vi "PJ1_ui-commu_1.vi"() -> ()   [LabVIEW 2024]
uses:
  contron/Control 7.ctl
  contron/Control 6.ctl
  contron/Control 5.ctl
  contron/Control 8.ctl
  contol_vr 23/66.ctl
  <vilib>/picture/picture.llb/imagedata.ctl
  contol_vr 23/Control 9.ctl
  contol_vr 23/6.ctl
  contol_vr 23/Control 4.ctl
  contol_vr 23/Control 3.ctl
  <vilib>/Instr/_visa.llb/VISA Configure Serial Port (Instr).vi
  <vilib>/express/express analysis/Spectral/Block/exnSpectralBlock spectral measurements PSD poly.vi
  <vilib>/express/express analysis/Spectral/Block/exnSpectralBlock spectral measurements PSD DDT.vi
  <vilib>/express/express analysis/Spectral/XNode/ExpressSpectralMeasurementsBlockNode.xnode
panel:
  out "check":bool
  out "Clear1":bool
  out "com":bool
  out "call":bool
  out "ele":bool
  in  "start":bool
  in  "Baseline":bool
  in  "VISA resource name":refnum<visa-resource-name>
  out "555":bool
  out "6 HZ 2":bool
  out "image data":T1
  out "7 HZ":bool
  in  "Upper Cut-Off":dbl=40.0
  out "PSD":dynamicdata(graph)
  out "PSD MAX":dbl
  out "Index ที่มากที่สุด":i32
  out "max value":dbl
  out "B 18+1":dbl
  out "N 18+1":dbl
  in  "Aj 18+1":dbl
  out "B 18+1":dbl
  out "PSD 18+1":dbl
  out "B 18":dbl
  out "N 18":dbl
  in  "Aj 18":dbl
  out "B 18":dbl
  out "PSD 18":dbl
  out "B 18-1":dbl
  out "N 18-1":dbl
  in  "Aj 18-1":dbl
  out "B 18-1":dbl
  out "PSD 18-1":dbl
  out "9 Hz":dbl[](array[numeric])
  out "Max Index 9":i32
  out "PSD max 9":dbl
  out "PSD 9-1":dbl
  out "B 9-1":dbl
  in  "Aj 9-1":dbl
  out "N 9-1":dbl
  out "B 9-1":dbl
  out "PSD 9":dbl
  out "B 9":dbl
  in  "Aj 9":dbl
  out "N 9":dbl
  out "B 9":dbl
  out "PSD 9+1":dbl
  out "B 9+1":dbl
  in  "Aj 9+1":dbl
  out "N 9+1":dbl
  out "B 9+1":dbl
  out "8 Hz":dbl[](array[numeric])
  out "Max Index 8":i32
  out "PSD max 8":dbl
  out "B 16+1":dbl
  out "N 16+1":dbl
  in  "Aj  16+1":dbl
  out "B 16+1":dbl
  out "PSD  16+1":dbl
  out "B 16":dbl
  out "N  16":dbl
  in  "Aj  16":dbl
  out "B 16":dbl
  out "PSD  16":dbl
  out "B 16-1":dbl
  out "N  16-1":dbl
  in  "Aj   16-1":dbl
  out "B   16-1":dbl
  out "PSD 16-1":dbl
  out "B 8+1":dbl
  out "N 8+1":dbl
  in  "Aj  8+1":dbl
  out "B  8+1":dbl
  out "PSD 8+1":dbl
  out "B 8":dbl
  out "N  8":dbl
  in  "Aj  8":dbl
  out "B  8":dbl
  out "PSD 8":dbl
  out "B 8-1":dbl
  out "N  8-1":dbl
  in  "Aj  8-1":dbl
  out "B  8-1":dbl
  out "PSD 8-1":dbl
  out "PSD 14+1":dbl
  out "B 14+1":dbl
  in  "Aj 14+1":dbl
  out "N 14+1":dbl
  out "B 14+1":dbl
  out "PSD 14":dbl
  out "B 14":dbl
  in  "Aj 14":dbl
  out "N 14":dbl
  out "B 14":dbl
  out "PSD 14-1":dbl
  out "B 14-1":dbl
  in  "Aj 14-1":dbl
  out "N 14-1":dbl
  out "B 14-1":dbl
  out "PSD7+1":dbl
  out "B7+1":dbl
  in  "Aj7+1":dbl
  out "N7+1":dbl
  out "B7+1":dbl
  out "PSD 7":dbl
  out "B 7":dbl
  in  "Aj 7":dbl
  out "N7":dbl
  out "B7":dbl
  out "7 Hz":dbl[](array[numeric])
  out "Max Index 7":i32
  out "PSD max 7":dbl
  out "PSD 7-1":dbl
  out "B 7-1":dbl
  in  "Aj 7-1":dbl
  out "N7-1":dbl
  out "B7-1":dbl
  out "B12-1":dbl
  out "N12-1":dbl
  in  "Aj 12-1":dbl
  out "B 12-1":dbl
  out "PSD 12-1":dbl
  out "B12":dbl
  out "N12":dbl
  in  "Aj 12":dbl
  out "B12":dbl
  out "PSD 12":dbl
  out "B12+1":dbl
  out "N12+1":dbl
  in  "Aj 12+1":dbl
  out "B 12+1":dbl
  out "PSD 12+1":dbl
  out "B6+1":dbl
  out "N6+1":dbl
  in  "Aj 6+1":dbl
  out "B 6+1":dbl
  out "PSD 6+1":dbl
  out "B6":dbl
  out "N6":dbl
  in  "Aj 6":dbl
  out "B6":dbl
  out "PSD 6":dbl
  out "PSD 6-1":dbl
  out "6 Hz":dbl[](array[numeric])
  out "Max Index 6":i32
  out "PSD max 6":dbl
  out "B 6-1":dbl
  in  "Aj 6-1":dbl
  out "N6-1":dbl
  out "B6-1":dbl
  out "appended array":dbl[][](array[numeric])
  out "Filtered Signal":dynamicdata(graph)
  in  "Lower Cut-Off":dbl=1.0
  out "data":dynamicdata(graph) caption="Raw Data"
  in  "number of samples":i32=1000
  in  "rate":dbl=200.0 min=200.0 max=200.0
  out "?":bool
  out "?":bool
  out "?":bool
  out "?":bool
  out "?":bool
  out "?":bool
  out "?":bool
  out "?":bool
  out "?":bool
  out "?":bool
  out "?":bool=TRUE
  out "?":bool=TRUE
  out "?":bool=TRUE
  out "?":bool=TRUE
  out "?":bool=TRUE
  out "?":bool=TRUE
  out "?":bool=TRUE
  out "?":bool=TRUE
  out "?":bool=TRUE
  out "?":bool=TRUE
  out "?":bool
  out "?":bool
  out "?":bool
  out "?":bool
  out "?":bool
  out "?":bool
  out "?":bool
  out "?":bool
  out "?":bool
  out "?":bool
  out "?":bool=TRUE
  out "?":bool=TRUE
  out "?":bool=TRUE
  out "?":bool=TRUE
  out "?":bool=TRUE
  out "?":bool=TRUE
  out "?":bool=TRUE
  out "?":bool=TRUE
  out "?":bool=TRUE
  out "?":bool=TRUE
  out "?":bool
  out "?":bool
  out "?":bool
  out "?":bool
  out "?":bool
  out "?":bool
  out "?":bool
  out "?":bool
  out "?":bool
  out "?":bool
  out "?":bool=TRUE
  out "?":bool=TRUE
  out "?":bool=TRUE
  out "?":bool=TRUE
  out "?":bool=TRUE
  out "?":bool=TRUE
  out "?":bool=TRUE
  out "?":bool=TRUE
  out "?":bool=TRUE
  out "?":bool=TRUE
  out "?":bool
  out "?":bool
  out "?":bool
  out "?":bool
  out "?":bool
  out "?":bool
  out "?":bool
  out "?":bool
  out "?":bool
  out "?":bool
  out "?":bool=TRUE
  out "?":bool=TRUE
  out "?":bool=TRUE
  out "?":bool=TRUE
  out "?":bool=TRUE
  out "?":bool=TRUE
  out "?":bool=TRUE
  out "?":bool=TRUE
  out "?":bool=TRUE
  out "?":bool=TRUE
  out "9 HZ":bool
  out "8 HZ":bool
  in  "Tab Control":T2(tab)
  out "Emotion 7":bool
  out "Emotion 6":bool
  out "Emotion 5":bool
  out "Emotion 4":bool
  out "ele":T3
  out "Emer":bool
  out "call":T4
  out "commu":T5
  in  "Activity":bool
  out "8-2":bool
  out "9-2":bool
  out "7-2":bool
  out "6-2":bool
  in  "Emotion":bool
  in  "ACC":T6
  in  "back_page2":T7
  in  "send":bool
  in  "BACK_Page3":bool
  out "Emotion 27":bool
  out "Emotion 26":bool
  out "Emotion 25":bool
  out "Emotion 24":bool
  in  "1 3":bool
  in  "1 2":T8
  in  "1":bool
  out "String 2":string
  in  "SOS CALLING":bool
  in  "Search Button 2":bool
  out "Emotion 15":bool
  out "Emotion 14":bool
  out "Emotion 13":bool
  out "Emotion 12":bool
  in  "Blank Button 14":bool
  in  "LED":bool
  in  "Blank Button 12":bool
  in  "BACK_Page4":bool
  out "BACK_page5":bool
  out "Emotion 3":bool
  out "Emotion 2":bool
  in  "BACK_Page5":bool=TRUE
  in  "Button 3":bool=TRUE
  in  "Button 2":bool=TRUE
  in  "Button 1":bool=TRUE
  out "Emotion 1":bool
  out "Emotion 11":bool
  in  "BACK_Page6":T9
  out "Emotion 10":bool
  out "Emotion 9":bool
  out "Emotion 8":bool
  in  "Activity 1":path
  out "new picture":picture
  in  "Activity 2":path
  in  "Activity 3":path
  out "new picture 2":picture
  out "new picture 3":picture
  out "Emotion 19":bool
  out "Emotion 18":bool
  out "Emotion 17":bool
  out "Emotion 16":bool
  out "new picture 7":picture
  in  "AAC13":path
  in  "Massage Send 3":string
  out "new picture 6":picture
  in  "AAC1 2":path
  in  "Massage Send 2":string
  out "new picture 5":picture
  in  "AAC1":path
  in  "BACK_Page7":bool
  in  "Massage Send 2":string
  out "Message Display":string
  in  "send 3":bool
  in  "Message Send":string
  in  "Clearpage 2":bool
  in  "Text3":T10
  in  "Text2":T11
  in  "Text1":bool
  in  "send 2":bool
  # "MENU"
  # "COMMUNICATION"
  # "SOS CALLING"
  # "Tel."
  # "ELECTRICAL DEVICES"
  # "EMOTIONS"
  # "ACTIVITIES"
  # "AAC"
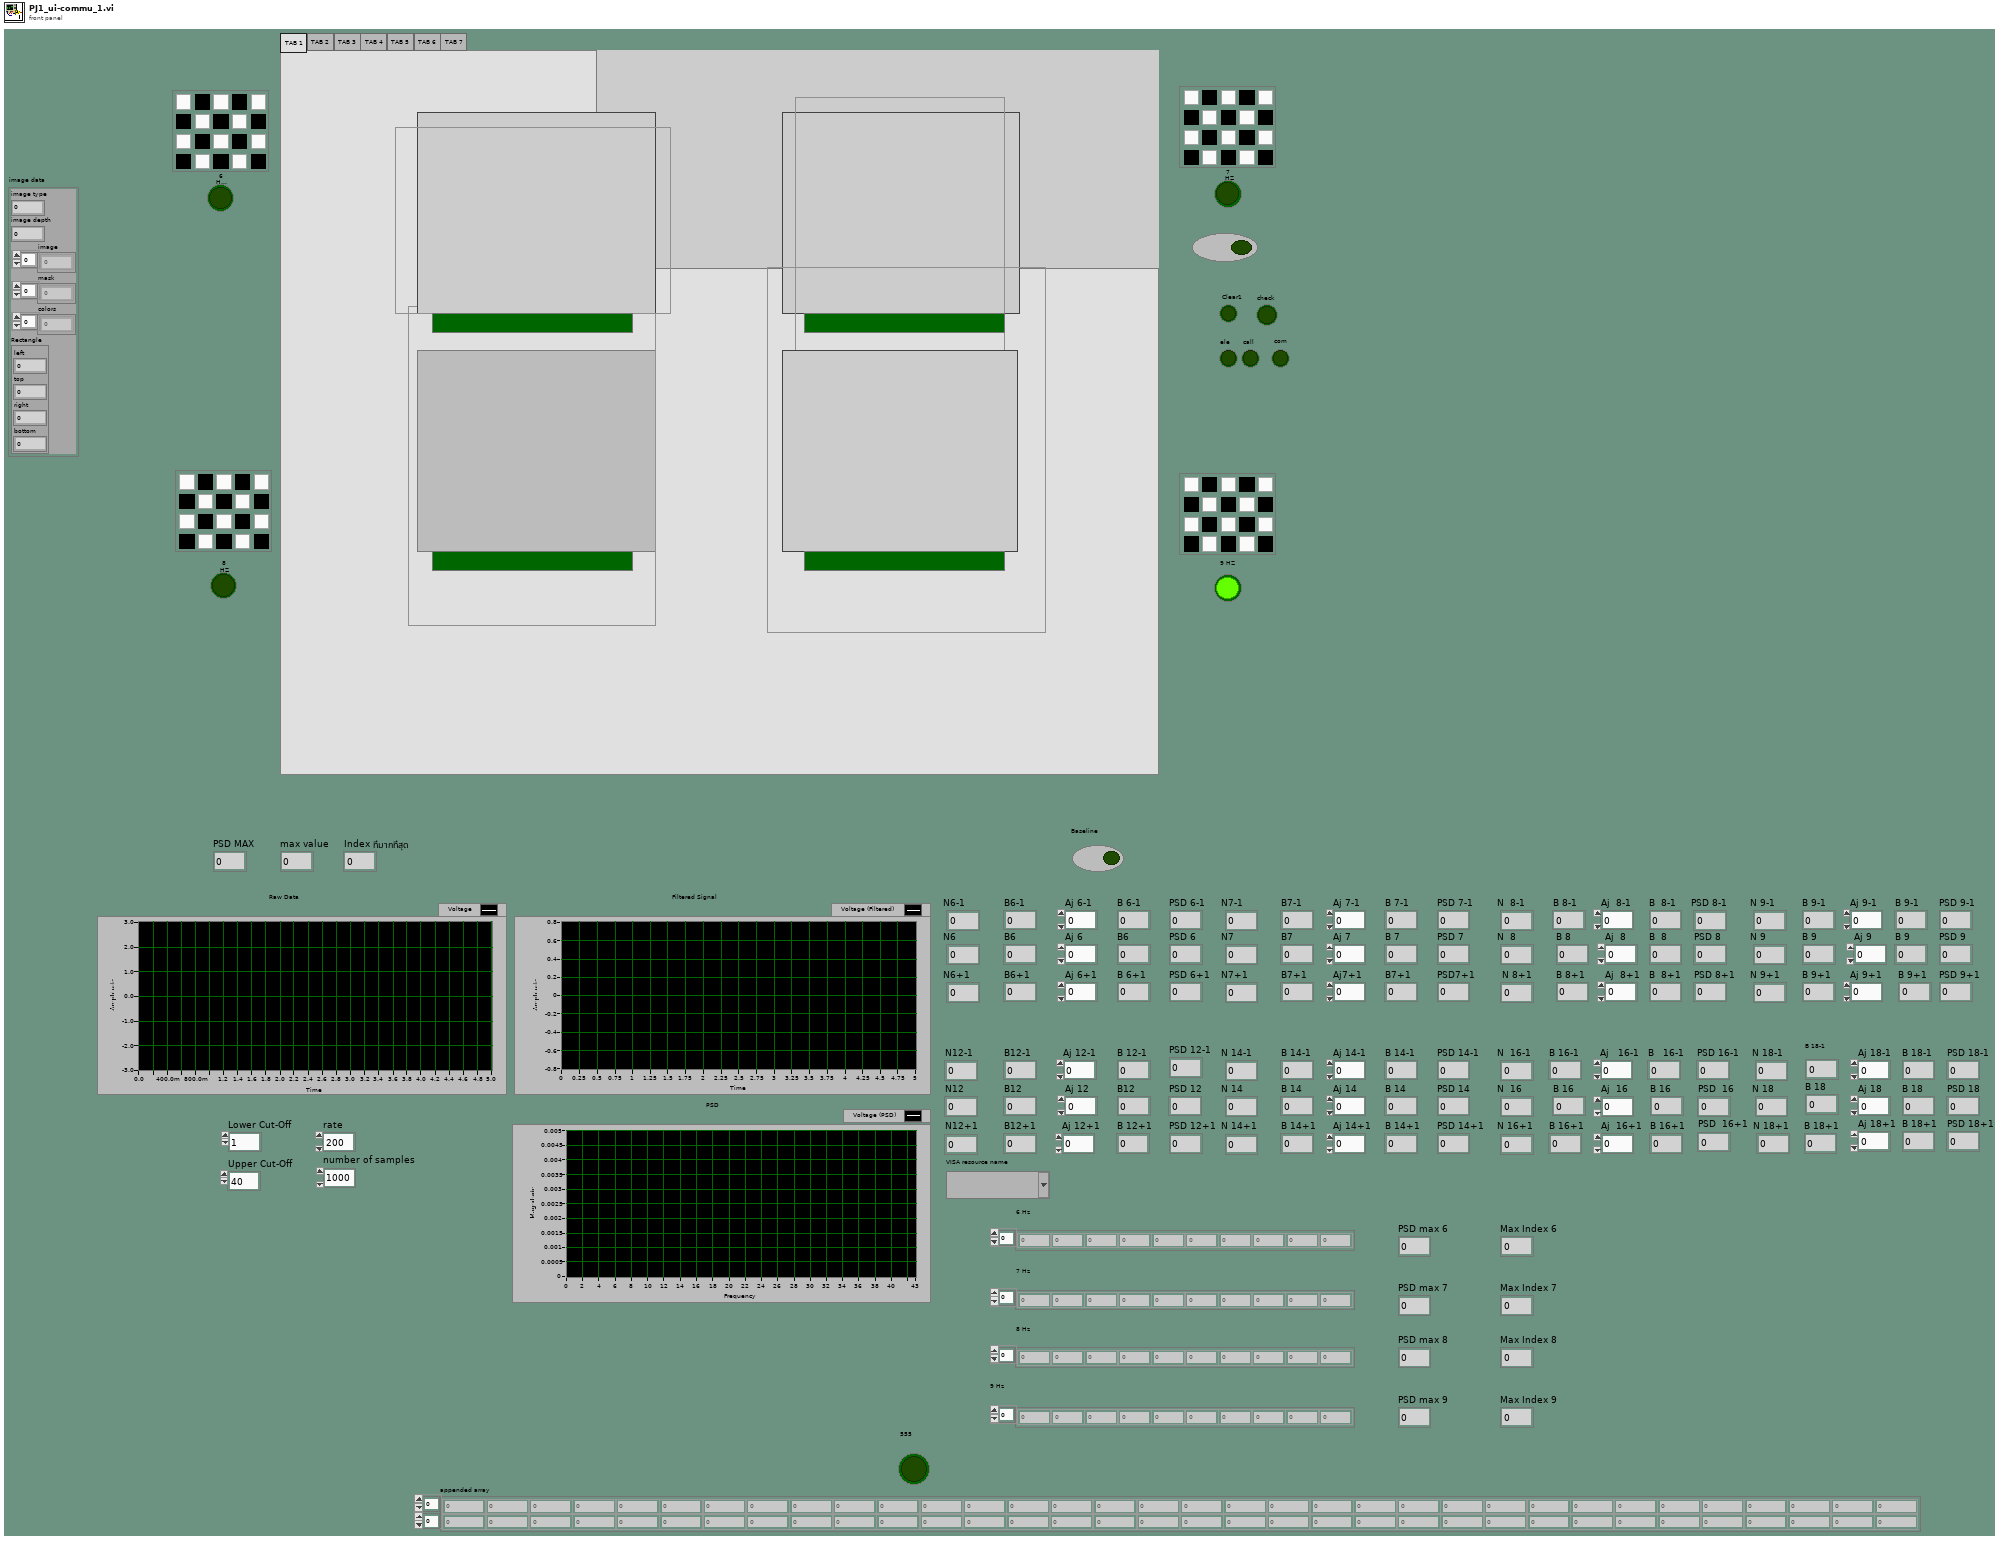
[diagram p1: front panel]
types:
  T1 = typedef "imagedata.ctl" = cluster{"image type":i32, "image depth":i32, "image":u8[], "mask":u8[], "colors":u32[], "Rectangle":cluster{"left":i16, "top":i16, "right":i16, "bottom":i16}}
  T2 = enum32{"TAB 1", "TAB 2", "TAB 3", "TAB 4", "TAB 5", "TAB 6", "TAB 7"}
  T3 = typedef "Control 5.ctl" = bool
  T4 = typedef "Control 6.ctl" = bool
  T5 = typedef "Control 7.ctl" = bool
  T6 = typedef "6.ctl" = bool
  T7 = typedef "66.ctl" = bool
  T8 = typedef "Control 8.ctl" = bool
  T9 = typedef "Control 9.ctl" = bool
  T10 = typedef "Control 4.ctl" = bool
  T11 = typedef "Control 3.ctl" = bool
  T12 = cluster{"averaging mode":u16, "weighting mode":u16, "number of averages":u32}
  T13 = cluster{"dB On (F)":bool, "unwrap phase (F)":bool, "convert to degree (F)":bool}
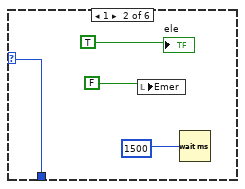
[diagram p2: hidden frame]
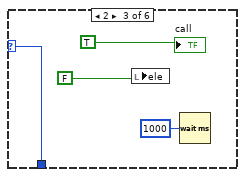
[diagram p3: hidden frame]
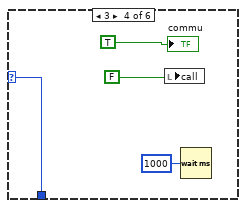
[diagram p4: hidden frame]
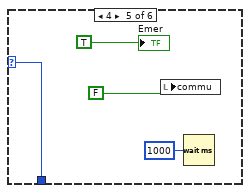
[diagram p5: hidden frame]
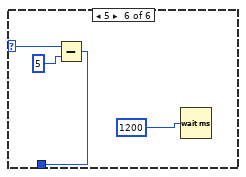
[diagram p6: hidden frame]
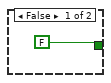
[diagram p8: hidden frame]
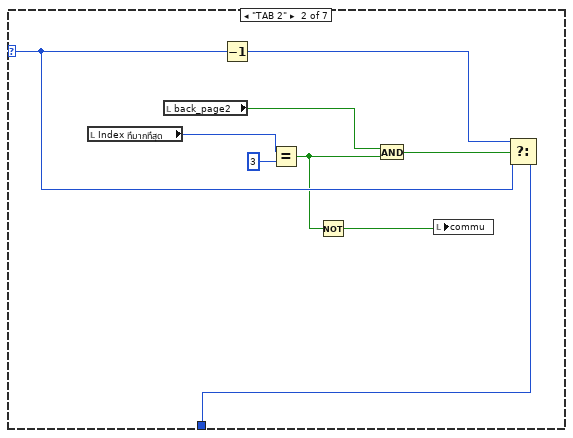
[diagram p9: hidden frame]
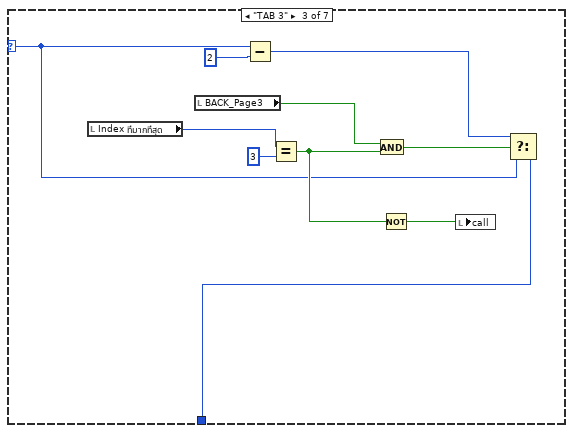
[diagram p10: hidden frame]
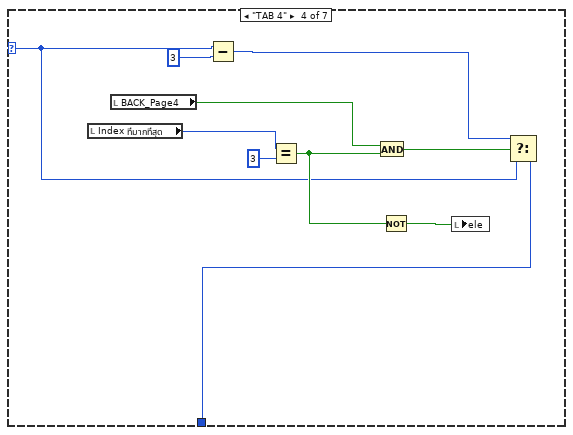
[diagram p11: hidden frame]
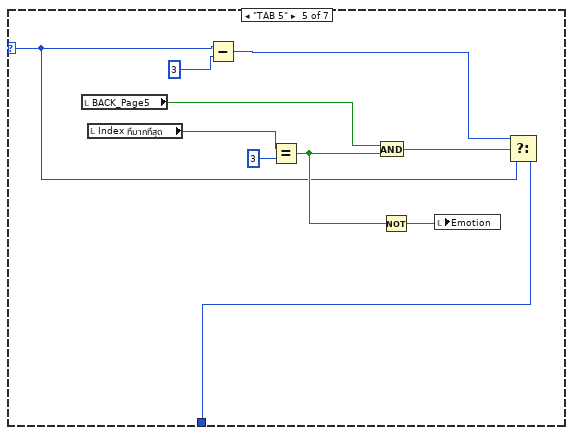
[diagram p12: hidden frame]
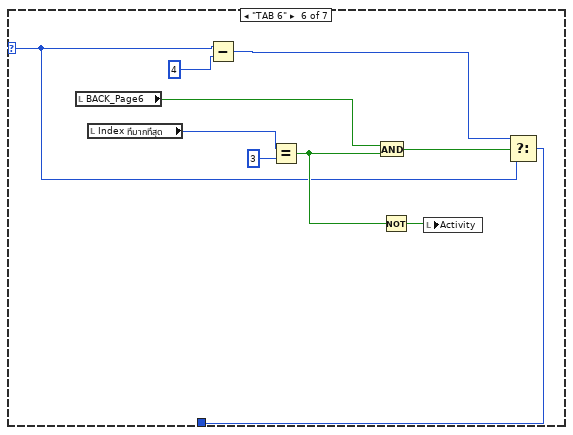
[diagram p13: hidden frame]
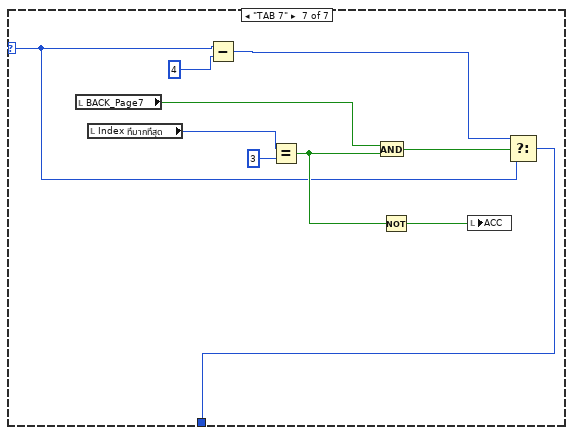
[diagram p14: hidden frame]
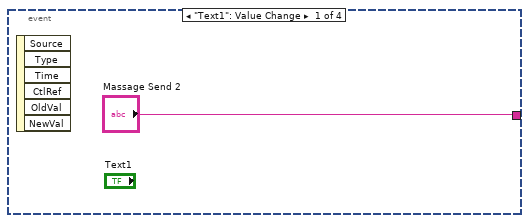
[diagram p15: hidden frame]
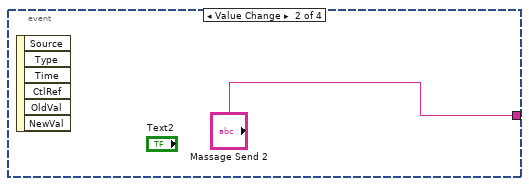
[diagram p16: hidden frame]
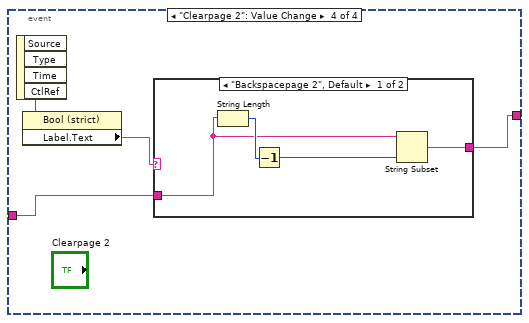
[diagram p17: hidden frame]
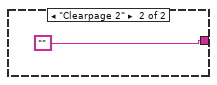
[diagram p18: hidden frame]
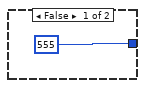
[diagram p19: hidden frame]
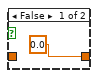
[diagram p20: hidden frame]
diagram:
  n1 = while {
    shift-right: [w23] -> _
    shift-left: "" -> [w25]
    stop <- FALSE stop-if-true
    n2 = event shown="[3] \"BACK_Page3\": Value Change" {
      selector: _ -> [_ _ _ _]
      dyn-events: _ -> [_ _ _ _]
      timeout: _ -> [_ _ _ _]
      tunnel: w25 -> [_ _ _ _]
      tunnel: ["0622436287" "1669" " 0937529340" _] -> w23
      event Value Change {
        n3 = event-data() -> ()  [unwired: 1 in, 6 out]
      }
      event "1": Value Change {
        n4 = event-data() -> ()  [unwired: 1 in, 6 out]
      }
      event "1 3": Value Change {
        n5 = event-data() -> ()  [unwired: 1 in, 6 out]
      }
      event "BACK_Page3": Value Change {
        n6 = event-data() -> ()  [unwired: 1 in, 6 out]
        n7 = local write "Tab Control"(enum32{"TAB 1", "TAB 2", "TAB 3", "TAB 4"}."TAB 1" ("Tab Control")) -> ()
      }
    }
    "String 2" <- w23
  }
  n8 = while {
    stop <- FALSE stop-if-true
    n9 = while {
      stop <- FALSE stop-if-true
      n10 = while {
        stop <- FALSE stop-if-true
        w69 = 83.3333
        # "6 HZ"
        n11 = for {
          N: 2 -> [_]
          tunnel: w69 -> [w73]
          i -> [w75]
          n12 = Wait (ms)(milliseconds to wait=w73) -> ()  [unwired: 1 out]
          n13 = Equal?(x=0, y=w75) -> (x = y?=→"?" →"?" →"?" →"?" →"?" →"?" →"?" →"?" →"?" →"?":bool)
        }
        n14 = for {
          N: 2 -> [_]
          tunnel: w69 -> [w77]
          i -> [w78]
          n15 = Wait (ms)(milliseconds to wait=w77) -> ()  [unwired: 1 out]
          n16 = Equal?(x=1, y=w78) -> (x = y?=→"?" →"?" →"?" →"?" →"?" →"?" →"?" →"?" →"?" →"?":bool)
        }
      }
      n17 = while {
        stop <- FALSE stop-if-true
        w57 = 71.428571
        # "7 HZ"
        n18 = for {
          N: 2 -> [_]
          tunnel: w57 -> [w61]
          i -> [w63]
          n19 = Wait (ms)(milliseconds to wait=w61) -> ()  [unwired: 1 out]
          n20 = Equal?(x=0, y=w63) -> (x = y?=→"?" →"?" →"?" →"?" →"?" →"?" →"?" →"?" →"?" →"?":bool)
        }
        n21 = for {
          N: 2 -> [_]
          tunnel: w57 -> [w65]
          i -> [w66]
          n22 = Wait (ms)(milliseconds to wait=w65) -> ()  [unwired: 1 out]
          n23 = Equal?(x=1, y=w66) -> (x = y?=→"?" →"?" →"?" →"?" →"?" →"?" →"?" →"?" →"?" →"?":bool)
        }
      }
      n24 = while {
        stop <- FALSE stop-if-true
        w45 = 62.5
        # "8 HZ"
        n25 = for {
          N: 2 -> [_]
          tunnel: w45 -> [w49]
          i -> [w51]
          n26 = Wait (ms)(milliseconds to wait=w49) -> ()  [unwired: 1 out]
          n27 = Equal?(x=0, y=w51) -> (x = y?=→"?" →"?" →"?" →"?" →"?" →"?" →"?" →"?" →"?" →"?":bool)
        }
        n28 = for {
          N: 2 -> [_]
          tunnel: w45 -> [w53]
          i -> [w54]
          n29 = Wait (ms)(milliseconds to wait=w53) -> ()  [unwired: 1 out]
          n30 = Equal?(x=1, y=w54) -> (x = y?=→"?" →"?" →"?" →"?" →"?" →"?" →"?" →"?" →"?" →"?":bool)
        }
      }
      n31 = while {
        stop <- FALSE stop-if-true
        w33 = 55.5555
        # "9 HZ"
        n32 = for {
          N: 2 -> [_]
          tunnel: w33 -> [w37]
          i -> [w39]
          n33 = Wait (ms)(milliseconds to wait=w37) -> ()  [unwired: 1 out]
          n34 = Equal?(x=0, y=w39) -> (x = y?=→"?" →"?" →"?" →"?" →"?" →"?" →"?" →"?" →"?" →"?":bool)
        }
        n35 = for {
          N: 2 -> [_]
          tunnel: w33 -> [w41]
          i -> [w42]
          n36 = Wait (ms)(milliseconds to wait=w41) -> ()  [unwired: 1 out]
          n37 = Equal?(x=1, y=w42) -> (x = y?=→"?" →"?" →"?" →"?" →"?" →"?" →"?" →"?" →"?" →"?":bool)
        }
      }
    }
  }
  n38 = while {
    stop <- FALSE stop-if-true
    n39 = call "DAQ Assistant2"("rate"="rate", "number of samples"="number of samples") -> ("data"=w84:dynamicdata)  [unwired: 15 in, 2 out]
    "data" <- w84
    n40 = Divide(x="rate", y="number of samples") -> (x/y=w171:dbl)
    n41 = call "Filter"("Lower Cut-Off"="Lower Cut-Off", "Upper Cut-Off"="Upper Cut-Off", "Signal"=w84) -> ("Filtered Signal"=w85:dynamicdata)  [unwired: 7 in, 1 out]
    "Filtered Signal" <- w85
    n42 = Divide(x=8.0, y=w171) -> (x/y=w271:dbl)
    n43 = Divide(x=16.0, y=w171) -> (x/y=w223:dbl)
    n44 = Divide(x=14.0, y=w171) -> (x/y=w296:dbl)
    n45 = Divide(x=18.0, y=w171) -> (x/y=w146:dbl)
    n46 = xnode "Spectral Measurements"("Signals"=w85) -> ("PSD"=w111:dynamicdata)  [unwired: 1 in, 1 out]
    "PSD" <- w111
    n47 = Divide(x=9.0, y=w171) -> (x/y=w189:dbl)
    n48 = Divide(x=7.0, y=w171) -> (x/y=w313:dbl)
    n49 = Divide(x=12.0, y=w171) -> (x/y=w382:dbl)
    n50 = Divide(x=6.0, y=w171) -> (x/y=w431:dbl)
    n51 = call "Convert from Dynamic Data"("Dynamic Data Type"=w111) -> ("Array"=w461:dbl[])  [unwired: 3 in]
    n52 = Decrement(x=w189) -> (x-1=w220:dbl)
    n53 = Increment(x=w189) -> (x+1=w188:dbl)
    n54 = Increment(x=w146) -> (x+1=w135:dbl)
    n55 = Decrement(x=w146) -> (x-1=w160:dbl)
    n56 = Decrement(x=w296) -> (x-1=w325:dbl)
    n57 = Increment(x=w271) -> (x+1=w261:dbl)
    n58 = Decrement(x=w223) -> (x-1=w246:dbl)
    n59 = Decrement(x=w431) -> (x-1=w444:dbl)
    n60 = Decrement(x=w313) -> (x-1=w354:dbl)
    "PSD 7-1" <- w354
    n61 = Increment(x=w313) -> (x+1=w339:dbl)
    n62 = Decrement(x=w271) -> (x-1=w284:dbl)
    n63 = Increment(x=w223) -> (x+1=w222:dbl)
    n64 = Increment(x=w431) -> (x+1=w420:dbl)
    n65 = Increment(x=w296) -> (x+1=w302:dbl)
    n66 = Decrement(x=w382) -> (x-1=w387:dbl)
    n67 = Increment(x=w382) -> (x+1=w381:dbl)
    n68 = Build Array(w461) -> (w136:dbl[][])
    "appended array" <- w136
    n69 = Index Array(array=w136, index (row)=0, index (col)=w246) -> (element=w257:dbl)
    "PSD 16-1" <- w257
    n70 = Index Array(array=w136, index (row)=0 ("disabled index (row)"), index (col)=w222) -> (element=w234:dbl)
    "PSD  16+1" <- w234
    n71 = Index Array(array=w136, index (row)=0 ("disabled index (row)"), index (col)=w223) -> (element=w236:dbl)
    "PSD  16" <- w236
    n72 = Index Array(array=w136, index (row)=0, index (col)=w302) -> (element=w303:dbl)
    "PSD 14+1" <- w303
    n73 = Index Array(array=w136, index (row)=0 ("disabled index (row)"), index (col)=w160) -> (element=w158:dbl)
    "PSD 18-1" <- w158
    n74 = Index Array(array=w136, index (row)=0, index (col)=w261) -> (element=w259:dbl)
    "PSD 8+1" <- w259
    n75 = Index Array(array=w136, index (row)=0 ("disabled index (row)"), index (col)=w135) -> (element=w132:dbl)
    "PSD 18+1" <- w132
    n76 = Index Array(array=w136, index (row)=0, index (col)=w188) -> (element=w177:dbl)
    "PSD 9-1" <- w177
    n77 = Index Array(array=w136, index (row)=0, index (col)=w271) -> (element=w282:dbl)
    "PSD 8" <- w282
    n78 = Index Array(array=w136, index (row)=0 ("disabled index (row)"), index (col)=w146) -> (element=w147:dbl)
    "PSD 18" <- w147
    n79 = Index Array(array=w136, index (row)=0, index (col)=w284) -> (element=w283:dbl)
    "PSD 8-1" <- w283
    n80 = Index Array(array=w136, index (row)=0, index (col)=w189) -> (element=w190:dbl)
    "PSD 9" <- w190
    n81 = Index Array(array=w136, index (row)=0, index (col)=w220) -> (element=w201:dbl)
    "PSD 9+1" <- w201
    n82 = Index Array(array=w136, index (row)=0, index (col)=w325) -> (element=w327:dbl)
    "PSD 14-1" <- w327
    n83 = Index Array(array=w136, index (row)=0, index (col)=w296) -> (element=w314:dbl)
    "PSD 14" <- w314
    n84 = Index Array(array=w136, index (row)=0, index (col)=w354) -> ()  [unwired: 1 out]
    n85 = Index Array(array=w136, index (row)=0 ("disabled index (row)"), index (col)=w313) -> (element=w351:dbl)
    "PSD 7" <- w351
    n86 = Index Array(array=w136, index (row)=0, index (col)=w339) -> (element=w340:dbl)
    "PSD7+1" <- w340
    n87 = Index Array(array=w136, index (row)=0 ("disabled index (row)"), index (col)=w420) -> (element=w418:dbl)
    "PSD 6+1" <- w418
    n88 = Index Array(array=w136, index (row)=0, index (col)=w387) -> (element=w386:dbl)
    "PSD 12-1" <- w386
    n89 = Index Array(array=w136, index (row)=0 ("disabled index (row)"), index (col)=w382) -> (element=w383:dbl)
    "PSD 12" <- w383
    n90 = Index Array(array=w136, index (row)=0 ("disabled index (row)"), index (col)=w381) -> (element=w379:dbl)
    "PSD 12+1" <- w379
    n91 = Index Array(array=w136, index (row)=0, index (col)=w431) -> (element=w432:dbl)
    "PSD 6" <- w432
    n92 = Index Array(array=w136, index (row)=0, index (col)=w444) -> (element=w451:dbl)
    "PSD 6-1" <- w451
    n93 = feedback #1() -> (w87:dbl)  [unwired: 1 in]
    "B 18" <- w87
    n94 = case shown="False" "Baseline" {
      tunnel: w147 -> [_ w472]
      tunnel: [w471 w472] -> w149
      tunnel: w87 -> [w471 _]
      frame False {
      }
      frame True {
      }
    }
    n95 = feedback-in #1(w149) -> ()
    n96 = feedback #2() -> (w88:dbl)  [unwired: 1 in]
    "B 18-1" <- w88
    n97 = case shown="False" "Baseline" {
      tunnel: w158 -> [_ w476]
      tunnel: [w475 w476] -> w169
      tunnel: w88 -> [w475 _]
      frame False {
      }
      frame True {
      }
    }
    n98 = feedback-in #2(w169) -> ()
    n99 = feedback #3() -> (w86:dbl)  [unwired: 1 in]
    "B 18+1" <- w86
    n100 = case shown="False" "Baseline" {
      tunnel: w132 -> [_ w468]
      tunnel: [w467 w468] -> w145
      tunnel: w86 -> [w467 _]
      frame False {
      }
      frame True {
      }
    }
    n101 = feedback-in #3(w145) -> ()
    n102 = feedback #4() -> (w94:dbl)  [unwired: 1 in]
    "B 16-1" <- w94
    n103 = case shown="True" "Baseline" {
      tunnel: w257 -> [_ w500]
      tunnel: [w499 w500] -> w247
      tunnel: w94 -> [w499 _]
      frame False {
      }
      frame True {
      }
    }
    n104 = feedback-in #4(w247) -> ()
    n105 = feedback #5() -> (w92:dbl)  [unwired: 1 in]
    "B 16+1" <- w92
    n106 = case shown="True" "Baseline" {
      tunnel: w234 -> [_ w492]
      tunnel: [w491 w492] -> w225
      tunnel: w92 -> [w491 _]
      frame False {
      }
      frame True {
      }
    }
    n107 = feedback-in #5(w225) -> ()
    n108 = feedback #6() -> (w93:dbl)  [unwired: 1 in]
    "B 16" <- w93
    n109 = case shown="True" "Baseline" {
      tunnel: w236 -> [_ w496]
      tunnel: [w495 w496] -> w245
      tunnel: w93 -> [w495 _]
      frame False {
      }
      frame True {
      }
    }
    n110 = feedback-in #6(w245) -> ()
    n111 = feedback #7() -> (w95:dbl)  [unwired: 1 in]
    "B 8+1" <- w95
    n112 = case shown="True" "Baseline" {
      tunnel: w259 -> [_ w504]
      tunnel: [w503 w504] -> w270
      tunnel: w95 -> [w503 _]
      frame False {
      }
      frame True {
      }
    }
    n113 = feedback-in #7(w270) -> ()
    n114 = feedback #8() -> (w98:dbl)  [unwired: 1 in]
    "B 14+1" <- w98
    n115 = case shown="True" "Baseline" {
      tunnel: w303 -> [_ w516]
      tunnel: [w515 w516] -> w304
      tunnel: w98 -> [w515 _]
      frame False {
      }
      frame True {
      }
    }
    n116 = feedback-in #8(w304) -> ()
    n117 = feedback #9() -> (w96:dbl)  [unwired: 1 in]
    "B 8" <- w96
    n118 = case shown="True" "Baseline" {
      tunnel: w282 -> [_ w508]
      tunnel: [w507 w508] -> w273
      tunnel: w96 -> [w507 _]
      frame False {
      }
      frame True {
      }
    }
    n119 = feedback-in #9(w273) -> ()
    n120 = feedback #10() -> (w90:dbl)  [unwired: 1 in]
    "B 9" <- w90
    n121 = case shown="False" "Baseline" {
      tunnel: w190 -> [_ w484]
      tunnel: [w483 w484] -> w191
      tunnel: w90 -> [w483 _]
      frame False {
      }
      frame True {
      }
    }
    n122 = feedback-in #10(w191) -> ()
    n123 = feedback #11() -> (w97:dbl)  [unwired: 1 in]
    "B 8-1" <- w97
    n124 = case shown="True" "Baseline" {
      tunnel: w283 -> [_ w512]
      tunnel: [w511 w512] -> w294
      tunnel: w97 -> [w511 _]
      frame False {
      }
      frame True {
      }
    }
    n125 = feedback-in #11(w294) -> ()
    n126 = feedback #12() -> (w91:dbl)  [unwired: 1 in]
    "B 9+1" <- w91
    n127 = case shown="True" "Baseline" {
      tunnel: w201 -> [_ w488]
      tunnel: [w487 w488] -> w202
      tunnel: w91 -> [w487 _]
      frame False {
      }
      frame True {
      }
    }
    n128 = feedback-in #12(w202) -> ()
    n129 = feedback #13() -> (w106:dbl)  [unwired: 1 in]
    "B12-1" <- w106
    n130 = case shown="True" "Baseline" {
      tunnel: w386 -> [_ w548]
      tunnel: [w547 w548] -> w398
      tunnel: w106 -> [w547 _]
      frame False {
      }
      frame True {
      }
    }
    n131 = feedback-in #13(w398) -> ()
    n132 = feedback #14() -> (w100:dbl)  [unwired: 1 in]
    "B 14-1" <- w100
    n133 = case shown="True" "Baseline" {
      tunnel: w327 -> [_ w524]
      tunnel: [w523 w524] -> w328
      tunnel: w100 -> [w523 _]
      frame False {
      }
      frame True {
      }
    }
    n134 = feedback-in #14(w328) -> ()
    n135 = feedback #15() -> (w89:dbl)  [unwired: 1 in]
    "B 9-1" <- w89
    n136 = case shown="False" "Baseline" {
      tunnel: w177 -> [_ w480]
      tunnel: [w479 w480] -> w178
      tunnel: w89 -> [w479 _]
      frame False {
      }
      frame True {
      }
    }
    n137 = feedback-in #15(w178) -> ()
    n138 = feedback #16() -> (w107:dbl)  [unwired: 1 in]
    "B6+1" <- w107
    n139 = case shown="True" "Baseline" {
      tunnel: w418 -> [_ w552]
      tunnel: [w551 w552] -> w421
      tunnel: w107 -> [w551 _]
      frame False {
      }
      frame True {
      }
    }
    n140 = feedback-in #16(w421) -> ()
    n141 = feedback #17() -> (w108:dbl)  [unwired: 1 in]
    "B6" <- w108
    n142 = case shown="True" "Baseline" {
      tunnel: w432 -> [_ w556]
      tunnel: [w555 w556] -> w442
      tunnel: w108 -> [w555 _]
      frame False {
      }
      frame True {
      }
    }
    n143 = feedback-in #17(w442) -> ()
    n144 = feedback #18() -> (w109:dbl)  [unwired: 1 in]
    "B6-1" <- w109
    n145 = case shown="False" "Baseline" {
      tunnel: w451 -> [_ w560]
      tunnel: [w559 w560] -> w443
      tunnel: w109 -> [w559 _]
      frame False {
      }
      frame True {
      }
    }
    n146 = feedback-in #18(w443) -> ()
    n147 = feedback #19() -> (w99:dbl)  [unwired: 1 in]
    "B 14" <- w99
    n148 = case shown="True" "Baseline" {
      tunnel: w314 -> [_ w520]
      tunnel: [w519 w520] -> w316
      tunnel: w99 -> [w519 _]
      frame False {
      }
      frame True {
      }
    }
    n149 = feedback-in #19(w316) -> ()
    n150 = feedback #20() -> (w104:dbl)  [unwired: 1 in]
    "B12+1" <- w104
    n151 = case shown="True" "Baseline" {
      tunnel: w379 -> [_ w540]
      tunnel: [w539 w540] -> w416
      tunnel: w104 -> [w539 _]
      frame False {
      }
      frame True {
      }
    }
    n152 = feedback-in #20(w416) -> ()
    n153 = Add(x=w87, y="Aj 18") -> (x+y=w153:dbl)
    "B 18" <- w153
    n154 = Add(x=w88, y="Aj 18-1") -> (x+y=w165:dbl)
    "B 18-1" <- w165
    n155 = Add(x=w86, y="Aj 18+1") -> (x+y=w141:dbl)
    "B 18+1" <- w141
    n156 = feedback #21() -> (w105:dbl)  [unwired: 1 in]
    "B12" <- w105
    n157 = case shown="True" "Baseline" {
      tunnel: w383 -> [_ w544]
      tunnel: [w543 w544] -> w399
      tunnel: w105 -> [w543 _]
      frame False {
      }
      frame True {
      }
    }
    n158 = feedback-in #21(w399) -> ()
    n159 = Add(x=w94, y="Aj   16-1") -> (x+y=w251:dbl)
    "B   16-1" <- w251
    n160 = Add(x=w92, y="Aj  16+1") -> (x+y=w229:dbl)
    "B 16+1" <- w229
    n161 = Add(x=w93, y="Aj  16") -> (x+y=w241:dbl)
    "B 16" <- w241
    n162 = Add(x=w95, y="Aj  8+1") -> (x+y=w266:dbl)
    "B  8+1" <- w266
    n163 = Add(x=w98, y="Aj 14+1") -> (x+y=w308:dbl)
    "B 14+1" <- w308
    n164 = Add(x=w96, y="Aj  8") -> (x+y=w277:dbl)
    "B  8" <- w277
    n165 = Add(x=w90, y="Aj 9") -> (x+y=w195:dbl)
    "B 9" <- w195
    n166 = Add(x=w97, y="Aj  8-1") -> (x+y=w290:dbl)
    "B  8-1" <- w290
    n167 = Add(x=w91, y="Aj 9+1") -> (x+y=w206:dbl)
    "B 9+1" <- w206
    n168 = Add(x=w106, y="Aj 12-1") -> (x+y=w394:dbl)
    "B 12-1" <- w394
    n169 = Add(x=w100, y="Aj 14-1") -> (x+y=w332:dbl)
    "B 14-1" <- w332
    n170 = Add(x=w89, y="Aj 9-1") -> (x+y=w182:dbl)
    "B 9-1" <- w182
    n171 = Multiply(x=w87, y=5.0) -> (x*y=w156:dbl)
    "N 18" <- w156
    n172 = Add(x=w107, y="Aj 6+1") -> (x+y=w425:dbl)
    "B 6+1" <- w425
    n173 = Multiply(x=w88, y=5.0) -> (x*y=w162:dbl)
    "N 18-1" <- w162
    n174 = Multiply(x=w86, y=5.0) -> (x*y=w138:dbl)
    "N 18+1" <- w138
    n175 = feedback #22() -> (w101:dbl)  [unwired: 1 in]
    "B7+1" <- w101
    n176 = case shown="True" "Baseline" {
      tunnel: w340 -> [_ w528]
      tunnel: [w527 w528] -> w342
      tunnel: w101 -> [w527 _]
      frame False {
      }
      frame True {
      }
    }
    n177 = feedback-in #22(w342) -> ()
    n178 = feedback #23() -> (w102:dbl)  [unwired: 1 in]
    "B7" <- w102
    n179 = case shown="True" "Baseline" {
      tunnel: w351 -> [_ w532]
      tunnel: [w531 w532] -> w355
      tunnel: w102 -> [w531 _]
      frame False {
      }
      frame True {
      }
    }
    n180 = feedback-in #23(w355) -> ()
    n181 = Multiply(x=w94, y=5.0) -> (x*y=w254:dbl)
    "N  16-1" <- w254
    n182 = Multiply(x=w92, y=5.0) -> (x*y=w232:dbl)
    "N 16+1" <- w232
    n183 = Multiply(x=w93, y=5.0) -> (x*y=w238:dbl)
    "N  16" <- w238
    n184 = Multiply(x=w95, y=5.0) -> (x*y=w263:dbl)
    "N 8+1" <- w263
    n185 = feedback #24() -> (w103:dbl)  [unwired: 1 in]
    "B7-1" <- w103
    n186 = case shown="True" "Baseline" {
      tunnel: w354 -> [_ w536]
      tunnel: [w535 w536] -> w368
      tunnel: w103 -> [w535 _]
      frame False {
      }
      frame True {
      }
    }
    n187 = feedback-in #24(w368) -> ()
    n188 = Add(x=w108, y="Aj 6") -> (x+y=w438:dbl)
    "B6" <- w438
    n189 = Add(x=w109, y="Aj 6-1") -> (x+y=w452:dbl)
    "B 6-1" <- w452
    n190 = Add(x=w99, y="Aj 14") -> (x+y=w320:dbl)
    "B 14" <- w320
    n191 = Multiply(x=w98, y=5.0) -> (x*y=w311:dbl)
    "N 14+1" <- w311
    n192 = Multiply(x=w96, y=5.0) -> (x*y=w280:dbl)
    "N  8" <- w280
    n193 = Multiply(x=w90, y=5.0) -> (x*y=w198:dbl)
    "N 9" <- w198
    n194 = Multiply(x=w97, y=5.0) -> (x*y=w287:dbl)
    "N  8-1" <- w287
    n195 = Multiply(x=w91, y=5.0) -> (x*y=w209:dbl)
    "N 9+1" <- w209
    n196 = Add(x=w104, y="Aj 12+1") -> (x+y=w412:dbl)
    "B 12+1" <- w412
    n197 = Multiply(x=w106, y=5.0) -> (x*y=w391:dbl)
    "N12-1" <- w391
    n198 = Multiply(x=w100, y=5.0) -> (x*y=w335:dbl)
    "N 14-1" <- w335
    n199 = Add(x=w105, y="Aj 12") -> (x+y=w403:dbl)
    "B12" <- w403
    n200 = Multiply(x=w89, y=5.0) -> (x*y=w185:dbl)
    "N 9-1" <- w185
    n201 = Multiply(x=w107, y=5.0) -> (x*y=w428:dbl)
    "N6+1" <- w428
    n202 = Greater?(x=w147, y=w153) -> (0:w154:bool)
    n203 = Greater?(x=w158, y=w165) -> (0:w164:bool)
    n204 = Greater?(x=w132, y=w141) -> (0:w140:bool)
    n205 = Less?(x=w147, y=w156) -> (x < y?=w155:bool)
    n206 = Less?(x=w158, y=w162) -> (x < y?=w163:bool)
    n207 = Multiply(x=w108, y=5.0) -> (x*y=w435:dbl)
    "N6" <- w435
    n208 = Multiply(x=w109, y=5.0) -> (x*y=w455:dbl)
    "N6-1" <- w455
    n209 = Multiply(x=w99, y=5.0) -> (x*y=w323:dbl)
    "N 14" <- w323
    n210 = Greater?(x=w257, y=w251) -> (0:w252:bool)
    n211 = Less?(x=w132, y=w138) -> (x < y?=w139:bool)
    n212 = Greater?(x=w234, y=w229) -> (0:w230:bool)
    n213 = Greater?(x=w236, y=w241) -> (0:w240:bool)
    n214 = Greater?(x=w259, y=w266) -> (0:w265:bool)
    n215 = Less?(x=w257, y=w254) -> (x < y?=w253:bool)
    n216 = Less?(x=w234, y=w232) -> (x < y?=w231:bool)
    n217 = Multiply(x=w104, y=5.0) -> (x*y=w409:dbl)
    "N12+1" <- w409
    n218 = Less?(x=w236, y=w238) -> (x < y?=w239:bool)
    n219 = Greater?(x=w303, y=w308) -> (0:w309:bool)
    n220 = Less?(x=w259, y=w263) -> (x < y?=w264:bool)
    n221 = Greater?(x=w282, y=w277) -> (0:w278:bool)
    n222 = Greater?(x=w190, y=w195) -> (0:w196:bool)
    n223 = Multiply(x=w105, y=5.0) -> (x*y=w406:dbl)
    "N12" <- w406
    n224 = Add(x=w101, y="Aj7+1") -> (x+y=w346:dbl)
    "B7+1" <- w346
    n225 = Less?(x=w303, y=w311) -> (x < y?=w310:bool)
    n226 = Greater?(x=w283, y=w290) -> (0:w289:bool)
    n227 = Less?(x=w282, y=w280) -> (x < y?=w279:bool)
    n228 = Less?(x=w190, y=w198) -> (x < y?=w197:bool)
    n229 = Greater?(x=w201, y=w206) -> (0:w207:bool)
    n230 = Add(x=w102, y="Aj 7") -> (x+y=w359:dbl)
    "B 7" <- w359
    n231 = Less?(x=w283, y=w287) -> (x < y?=w288:bool)
    n232 = Greater?(x=w386, y=w394) -> (0:w393:bool)
    n233 = Greater?(x=w327, y=w332) -> (0:w333:bool)
    n234 = Less?(x=w201, y=w209) -> (x < y?=w208:bool)
    n235 = Greater?(x=w177, y=w182) -> (0:w183:bool)
    n236 = Add(x=w103, y="Aj 7-1") -> (x+y=w372:dbl)
    "B 7-1" <- w372
    n237 = Greater?(x=w418, y=w425) -> (0:w426:bool)
    n238 = Less?(x=w386, y=w391) -> (x < y?=w392:bool)
    n239 = Less?(x=w327, y=w335) -> (x < y?=w334:bool)
    n240 = Less?(x=w177, y=w185) -> (x < y?=w184:bool)
    n241 = Less?(x=w418, y=w428) -> (x < y?=w427:bool)
    n242 = And(x=w155, y=w154) -> (x .and. y?=w152:bool)
    n243 = Subtract(x=w147, y=w153) -> (x-y=w151:dbl)
    n244 = And(x=w163, y=w164) -> (x .and. y?=w166:bool)
    n245 = Greater?(x=w432, y=w438) -> (0:w437:bool)
    n246 = Subtract(x=w158, y=w165) -> (x-y=w167:dbl)
    n247 = Greater?(x=w451, y=w452) -> (0:w453:bool)
    n248 = Greater?(x=w314, y=w320) -> (0:w321:bool)
    n249 = And(x=w139, y=w140) -> (x .and. y?=w142:bool)
    n250 = Subtract(x=w132, y=w141) -> (x-y=w143:dbl)
    n251 = Less?(x=w432, y=w435) -> (x < y?=w436:bool)
    n252 = Less?(x=w451, y=w455) -> (x < y?=w454:bool)
    n253 = Less?(x=w314, y=w323) -> (x < y?=w322:bool)
    n254 = And(x=w253, y=w252) -> (x .and. y?=w250:bool)
    n255 = Multiply(x=w101, y=5.0) -> (x*y=w349:dbl)
    "N7+1" <- w349
    n256 = Subtract(x=w257, y=w251) -> (x-y=w249:dbl)
    n257 = And(x=w231, y=w230) -> (x .and. y?=w228:bool)
    n258 = Subtract(x=w234, y=w229) -> (x-y=w227:dbl)
    n259 = Greater?(x=w379, y=w412) -> (0:w411:bool)
    n260 = Multiply(x=w102, y=5.0) -> (x*y=w362:dbl)
    "N7" <- w362
    n261 = And(x=w239, y=w240) -> (x .and. y?=w242:bool)
    n262 = And(x=w264, y=w265) -> (x .and. y?=w267:bool)
    n263 = Subtract(x=w236, y=w241) -> (x-y=w243:dbl)
    n264 = Subtract(x=w259, y=w266) -> (x-y=w268:dbl)
    n265 = Greater?(x=w383, y=w403) -> (0:w404:bool)
    n266 = Less?(x=w379, y=w409) -> (x < y?=w410:bool)
    n267 = And(x=w310, y=w309) -> (x .and. y?=w307:bool)
    n268 = Subtract(x=w303, y=w308) -> (x-y=w306:dbl)
    n269 = Multiply(x=w103, y=5.0) -> (x*y=w375:dbl)
    "N7-1" <- w375
    n270 = And(x=w279, y=w278) -> (x .and. y?=w276:bool)
    n271 = Subtract(x=w282, y=w277) -> (x-y=w275:dbl)
    n272 = And(x=w197, y=w196) -> (x .and. y?=w194:bool)
    n273 = Subtract(x=w190, y=w195) -> (x-y=w193:dbl)
    n274 = Less?(x=w383, y=w406) -> (x < y?=w405:bool)
    n275 = And(x=w288, y=w289) -> (x .and. y?=w291:bool)
    n276 = Subtract(x=w283, y=w290) -> (x-y=w292:dbl)
    n277 = And(x=w208, y=w207) -> (x .and. y?=w205:bool)
    n278 = Subtract(x=w201, y=w206) -> (x-y=w204:dbl)
    n279 = And(x=w392, y=w393) -> (x .and. y?=w395:bool)
    n280 = Subtract(x=w386, y=w394) -> (x-y=w396:dbl)
    n281 = And(x=w334, y=w333) -> (x .and. y?=w331:bool)
    n282 = Subtract(x=w327, y=w332) -> (x-y=w330:dbl)
    n283 = And(x=w184, y=w183) -> (x .and. y?=w181:bool)
    n284 = Subtract(x=w177, y=w182) -> (x-y=w180:dbl)
    n285 = Subtract(x=w418, y=w425) -> (x-y=w423:dbl)
    n286 = And(x=w427, y=w426) -> (x .and. y?=w424:bool)
    n287 = And(x=w454, y=w453) -> (x .and. y?=w450:bool)
    n288 = Subtract(x=w432, y=w438) -> (x-y=w440:dbl)
    n289 = And(x=w322, y=w321) -> (x .and. y?=w319:bool)
    n290 = Subtract(x=w451, y=w452) -> (x-y=w449:dbl)
    n291 = Greater?(x=w340, y=w346) -> (0:w347:bool)
    n292 = Subtract(x=w314, y=w320) -> (x-y=w318:dbl)
    n293 = Greater?(x=w351, y=w359) -> (0:w360:bool)
    n294 = And(x=w436, y=w437) -> (x .and. y?=w439:bool)
    n295 = Less?(x=w340, y=w349) -> (x < y?=w348:bool)
    n296 = Less?(x=w351, y=w362) -> (x < y?=w361:bool)
    n297 = Subtract(x=w379, y=w412) -> (x-y=w414:dbl)
    n298 = Greater?(x=w354, y=w372) -> (0:w373:bool)
    n299 = Subtract(x=w383, y=w403) -> (x-y=w401:dbl)
    n300 = And(x=w410, y=w411) -> (x .and. y?=w413:bool)
    n301 = Less?(x=w354, y=w375) -> (x < y?=w374:bool)
    n302 = And(x=w405, y=w404) -> (x .and. y?=w402:bool)
    n303 = And(x=w348, y=w347) -> (x .and. y?=w345:bool)
    n304 = Subtract(x=w340, y=w346) -> (x-y=w344:dbl)
    n305 = And(x=w361, y=w360) -> (x .and. y?=w358:bool)
    n306 = Subtract(x=w351, y=w359) -> (x-y=w357:dbl)
    n307 = And(x=w374, y=w373) -> (x .and. y?=w371:bool)
    n308 = Subtract(x=w354, y=w372) -> (x-y=w370:dbl)
    n309 = case shown="True" w395 {
      tunnel: w396 -> [_ w546]
      tunnel: [0.0 w546] -> w385
      frame False {
      }
      frame True {
      }
    }
    n310 = case shown="True" w424 {
      tunnel: w423 -> [_ w550]
      tunnel: [0.0 w550] -> w417
      frame False {
      }
      frame True {
      }
    }
    n311 = case shown="False" w450 {
      tunnel: w449 -> [_ w558]
      tunnel: [0.0 w558] -> w447
      frame False {
      }
      frame True {
      }
    }
    n312 = case shown="False" w439 {
      tunnel: w440 -> [_ w554]
      tunnel: [0.0 w554] -> w430
      frame False {
      }
      frame True {
      }
    }
    n313 = case shown="True" w413 {
      tunnel: w414 -> [_ w538]
      tunnel: [0.0 w538] -> w377
      frame False {
      }
      frame True {
      }
    }
    n314 = case shown="True" w152 {
      tunnel: w151 -> [_ w470]
      tunnel: [0.0 w470] -> w130
      frame False {
      }
      frame True {
      }
    }
    n315 = case shown="True" w402 {
      tunnel: w401 -> [_ w542]
      tunnel: [0.0 w542] -> w378
      frame False {
      }
      frame True {
      }
    }
    n316 = case shown="True" w166 {
      tunnel: w167 -> [_ w474]
      tunnel: [0.0 w474] -> w131
      frame False {
      }
      frame True {
      }
    }
    n317 = case shown="True" w142 {
      tunnel: w143 -> [_ w466]
      tunnel: [0.0 w466] -> w129
      frame False {
      }
      frame True {
      }
    }
    n318 = case shown="True" w250 {
      tunnel: w249 -> [_ w498]
      tunnel: [0.0 w498] -> w213
      frame False {
      }
      frame True {
      }
    }
    n319 = case shown="True" w228 {
      tunnel: w227 -> [_ w490]
      tunnel: [0.0 w490] -> w211
      frame False {
      }
      frame True {
      }
    }
    n320 = case shown="True" w242 {
      tunnel: w243 -> [_ w494]
      tunnel: [0.0 w494] -> w212
      frame False {
      }
      frame True {
      }
    }
    n321 = case shown="True" w267 {
      tunnel: w268 -> [_ w502]
      tunnel: [0.0 w502] -> w214
      frame False {
      }
      frame True {
      }
    }
    n322 = case shown="True" w307 {
      tunnel: w306 -> [_ w514]
      tunnel: [0.0 w514] -> w298
      frame False {
      }
      frame True {
      }
    }
    n323 = case shown="True" w276 {
      tunnel: w275 -> [_ w506]
      tunnel: [0.0 w506] -> w215
      frame False {
      }
      frame True {
      }
    }
    n324 = case shown="True" w319 {
      tunnel: w318 -> [_ w518]
      tunnel: [0.0 w518] -> w299
      frame False {
      }
      frame True {
      }
    }
    n325 = case shown="True" w194 {
      tunnel: w193 -> [_ w482]
      tunnel: [0.0 w482] -> w173
      frame False {
      }
      frame True {
      }
    }
    n326 = case shown="True" w291 {
      tunnel: w292 -> [_ w510]
      tunnel: [0.0 w510] -> w216
      frame False {
      }
      frame True {
      }
    }
    n327 = case shown="True" w331 {
      tunnel: w330 -> [_ w522]
      tunnel: [0.0 w522] -> w300
      frame False {
      }
      frame True {
      }
    }
    n328 = case shown="True" w345 {
      tunnel: w344 -> [_ w526]
      tunnel: [0.0 w526] -> w337
      frame False {
      }
      frame True {
      }
    }
    n329 = case shown="True" w205 {
      tunnel: w204 -> [_ w486]
      tunnel: [0.0 w486] -> w174
      frame False {
      }
      frame True {
      }
    }
    n330 = case shown="True" w358 {
      tunnel: w357 -> [_ w530]
      tunnel: [0.0 w530] -> w338
      frame False {
      }
      frame True {
      }
    }
    n331 = case shown="True" w181 {
      tunnel: w180 -> [_ w478]
      tunnel: [0.0 w478] -> w172
      frame False {
      }
      frame True {
      }
    }
    n332 = case shown="False" w371 {
      tunnel: w370 -> [_ w534]
      tunnel: [0.0 w534] -> w364
      frame False {
      }
      frame True {
      }
    }
    n333 = Build Array(w364, w338, w337, w300, w299, w298) -> (w365:dbl[])
    "7 Hz" <- w365
    n334 = Build Array(w447, w430, w417, w385, w378, w377) -> (w445:dbl[])
    "6 Hz" <- w445
    n335 = Array Max & Min(array=w365) -> (max value=w128:dbl, max index (indices)=→"Max Index 7":i32)  [unwired: 2 out]
    "PSD max 7" <- w128
    n336 = Array Max & Min(array=w445) -> (max value=w125:dbl, max index (indices)=→"Max Index 6":i32)  [unwired: 2 out]
    "PSD max 6" <- w125
    n337 = Build Array(w216, w215, w214, w213, w212, w211) -> (w217:dbl[])
    "8 Hz" <- w217
    n338 = Build Array(w174, w173, w172, w131, w130, w129) -> (w175:dbl[])
    "9 Hz" <- w175
    n339 = Array Max & Min(array=w217) -> (max value=w127:dbl, max index (indices)=→"Max Index 8":i32)  [unwired: 2 out]
    "PSD max 8" <- w127
    n340 = Array Max & Min(array=w175) -> (max value=w126:dbl, max index (indices)=→"Max Index 9":i32)  [unwired: 2 out]
    "PSD max 9" <- w126
    n341 = Build Array(w125, w128, w127, w126) -> (w124:dbl[])
    n342 = Array Max & Min(array=w124) -> (max value=w122:dbl, max index (indices)=w123:i32)  [unwired: 2 out]
    "max value" <- w122
    "PSD MAX" <- w122
    n343 = Greater?(x=w122, y=0.0 ("x")) -> (0:w120:bool)
    n344 = case shown="True" w120 {
      tunnel: w123 -> [_ w464]
      tunnel: [555 w464] -> w112
      frame False {
      }
      frame True {
      }
    }
    "Index ที่มากที่สุด" <- w112
    n345 = Equal?(x=0, y=w112) -> (x = y?=→"6 HZ 2" →"Emotion 4" →"6-2" →"Emotion 8" →"Emotion 16" →"Emotion 24":bool)
    n346 = Equal?(x=1, y=w112) -> (x = y?=→"7 HZ" →"Emotion 5" →"7-2" →"Emotion 9" →"Emotion 17" →"Emotion 25":bool)
    n347 = Equal?(x=2, y=w112) -> (x = y?=→"8 HZ" →"Emotion 6" →"8-2" →"Emotion 10" →"Emotion 19" →"Emotion 27":bool)
    n348 = Equal?(x=3, y=w112) -> (x = y?=→"9 HZ" →"Emotion 7" →"9-2" →"Emotion 11" →"Emotion 18" →"Emotion 26":bool)
    n349 = Equal?(x=555, y=w112) -> (x = y?=→"555":bool)
  }
  n350 = while {
    stop <- FALSE stop-if-true
    n351 = event shown="[4] \"Emer\": Value Change" {
      selector: _ -> [_ _ _ _ _ _ _]
      dyn-events: _ -> [_ _ _ _ _ _ _]
      timeout: _ -> [_ _ _ _ _ _ _]
      event Timeout {
        n352 = event-data() -> ()  [unwired: 1 in, 3 out]
      }
      event Value Change {
        n353 = event-data() -> ()  [unwired: 1 in, 6 out]
        n354 = local write "Tab Control"(enum32{"TAB 1", "TAB 2", "TAB 3", "TAB 4"}."TAB 2" ("Tab Control")) -> ()
      }
      event Value Change {
        n355 = event-data() -> ()  [unwired: 1 in, 6 out]
        n356 = local write "Tab Control"(enum32{"TAB 1", "TAB 2", "TAB 3", "TAB 4"}."TAB 3" ("Tab Control")) -> ()
      }
      event Value Change {
        n357 = event-data() -> ()  [unwired: 1 in, 6 out]
        n358 = local write "Tab Control"(T2."TAB 1" ("Tab Control")) -> ()
      }
      event "Emer": Value Change {
        n359 = event-data() -> ()  [unwired: 1 in, 6 out]
        n360 = local write "Tab Control"(enum32{"TAB 1", "TAB 2", "TAB 3", "TAB 4"}."TAB 4" ("Tab Control")) -> ()
      }
      event Value Change {
        n361 = event-data() -> ()  [unwired: 1 in, 6 out]
        n362 = local write "Tab Control"(enum32{"TAB 1", "TAB 2", "TAB 3", "TAB 4"}."TAB 4" ("Tab Control")) -> ()
      }
      event "BACK_Page4": Value Change {
        n363 = event-data() -> ()  [unwired: 1 in, 6 out]
        n364 = local write "Tab Control"(enum32{"TAB 1", "TAB 2", "TAB 3", "TAB 4"}."TAB 1" ("Tab Control")) -> ()
      }
    }
  }
  n365 = call-poly "VISA Configure Serial Port"("VISA resource name"="VISA resource name", "baud rate (9600)"=u32 9600) -> ("VISA resource name out"=w22:refnum<visa-resource-name>, "error out"=w20:errorcluster)  [unwired: 12 in]
  n366 = while {
    shift-right: [w585] -> w21
    shift-left: w22 -> [w586]
    shift-right: [w583] -> w19
    shift-left: w20 -> [w584]
    stop <- FALSE stop-if-true
    n367 = Select(t="a", s="LED", f="b") -> (s? t:f=w580:string)
    n368 = VISA Write(VISA resource name=w586, write buffer=w580, error in (no error)=w584) -> (VISA resource name out=w585:refnum<visa-resource-name>, error out=w583:errorcluster)  [unwired: 1 out]
    n369 = Wait (ms)(milliseconds to wait=u32 5) -> ()  [unwired: 1 out]
  }
  n370 = VISA Close(VISA resource name=w21, error in (no error)=w19) -> ()  [unwired: 1 out]
  n371 = call <vilib>:"Read JPEG File.vi"("path to JPEG file"="Activity 1") -> ("image data"=w13:T1)  [unwired: 8 in, 2 out]
  "image data" <- w13
  n372 = call <vilib>:"Read JPEG File.vi"("path to JPEG file"="Activity 3") -> ("image data"=w7:T1)  [unwired: 8 in, 2 out]
  n373 = call <vilib>:"Read JPEG File.vi"("path to JPEG file"="Activity 2") -> ("image data"=w12:T1)  [unwired: 8 in, 2 out]
  n374 = call <vilib>:"Draw Flattened Pixmap.vi"("image data"=w13) -> ("new picture"=→"new picture":picture)  [unwired: 8 in]
  n375 = call <vilib>:"Draw Flattened Pixmap.vi"("image data"=w7) -> ("new picture"=→"new picture 3":picture)  [unwired: 8 in]
  n376 = call <vilib>:"Draw Flattened Pixmap.vi"("image data"=w12) -> ("new picture"=→"new picture 2":picture)  [unwired: 8 in]
  n377 = local read "Tab Control"() -> (w2:T2)
  n378 = Obtain Notifier(notification data type=w2) -> (notifier out=w1:refnum<notifier>, error out=w4:errorcluster)  [unwired: 3 in, 1 out]
  n379 = while {
    tunnel: w1 -> [w588]
    stop <- FALSE stop-if-true
    n380 = Wait on Notification(notifier=w588) -> (notification=w587:T2)  [unwired: 3 in, 3 out]
    n381 = case shown="\"TAB 1\"" w587 {
      frame "TAB 1" {
        n382 = while {
          stop <- w638 stop-if-true
          n383 = case shown="True" "start" {
            tunnel: [FALSE ("check") w680] -> w652
            frame False {
            }
            frame True {
              n384 = local read "start"() -> (w680:bool)
            }
          }
          n385 = feedback #25() -> (w650:i32)  [unwired: 1 in]
          n386 = case shown="True" w652 {
            tunnel: [w676 w677] -> w651
            tunnel: w650 -> [w676 w678]
            frame False {
            }
            frame True {
              n387 = Increment(x=w678) -> (x+1=w677:i32)
            }
          }
          n388 = case shown="0, Default" w651 {
            selector: w651 -> [w655 w659 w660 w667 w671 w674]
            tunnel: [w655 w659 w660 w667 w671 w673] -> w649
            frame 0, Default {
              w654 = FALSE ("B")
              n389 = local write "ele"(w654) -> ()
              n390 = local write "call"(w654) -> ()
              n391 = local write "commu"(w654) -> ()
              n392 = local write "Emotion"(w654) -> ()
              n393 = local write "Activity"(w654) -> ()
              n394 = local write "ACC"(w654) -> ()
            }
            frame 1 {
              n395 = local write "Emer"(FALSE) -> ()
              n396 = Wait (ms)(milliseconds to wait=u32 1500 ("millisecond timer value")) -> ()  [unwired: 1 out]
              "ele" <- TRUE
            }
            frame 2 {
              n397 = local write "ele"(FALSE) -> ()
              n398 = Wait (ms)(milliseconds to wait=u32 1000) -> ()  [unwired: 1 out]
              "call" <- TRUE
            }
            frame 3 {
              n399 = local write "call"(FALSE) -> ()
              n400 = Wait (ms)(milliseconds to wait=u32 1000) -> ()  [unwired: 1 out]
              "commu" <- TRUE
            }
            frame 4 {
              n401 = local write "commu"(FALSE) -> ()
              n402 = Wait (ms)(milliseconds to wait=u32 1000) -> ()  [unwired: 1 out]
              "Emer" <- TRUE
            }
            frame 5 {
              n403 = Subtract(x=w674, y=5 ("x")) -> (x-y=w673:i32)
              n404 = Wait (ms)(milliseconds to wait=u32 1200 ("millisecond timer value")) -> ()  [unwired: 1 out]
            }
          }
          n405 = feedback-in #25(w649) -> ()
          n406 = local read "Tab Control"() -> (w640:T2)
          n407 = Equal?(x=w640, y=T2."TAB 2" ("Tab Control")) -> (x = y?=w648:bool)
          n408 = Equal?(x=w640, y=T2."TAB 6" ("Tab Control")) -> (x = y?=w642:bool)
          n409 = Equal?(x=w640, y=T2."TAB 3" ("Tab Control")) -> (x = y?=w647:bool)
          n410 = Equal?(x=w640, y=T2."TAB 4" ("Tab Control")) -> (x = y?=w646:bool)
          n411 = Equal?(x=w640, y=T2."TAB 7" ("Tab Control")) -> (x = y?=w641:bool)
          n412 = Equal?(x=w640, y=T2."TAB 5" ("Tab Control")) -> (x = y?=w645:bool)
          n413 = Or(x=w648, y=w647) -> (x .or. y?=w644:bool)
          n414 = Or(x=w642, y=w641) -> (x .or. y?=w637:bool)
          n415 = Or(x=w646, y=w645) -> (x .or. y?=w643:bool)
          n416 = Or(x=w644, y=w643) -> (x .or. y?=w639:bool)
          n417 = Or(x=w639, y=w637) -> (x .or. y?=w638:bool)
        }
        n418 = while {
          stop <- w609 stop-if-true
          n419 = flat-sequence {
            frame #0 {
              n420 = while {
                stop <- w612 stop-if-true
                n421 = local read "Clear1"() -> (w610:bool)
                n422 = local read "ele"() -> (w611:T3)
                n423 = Or(x=w611, y=w610) -> (x .or. y?=w612:T3)
              }
            }
            frame #1 {
              n424 = while {
                stop <- w618 stop-if-true
                n425 = local read "Index ที่มากที่สุด"() -> (w617:i32)
                n426 = local read "Clear1"() -> (w613:bool)
                n427 = local read "call"() -> (w615:T4)
                n428 = Equal?(x=w617, y=0) -> (x = y?=→"ele":bool)
                n429 = Or(x=w615, y=w613) -> (x .or. y?=w618:T4)
              }
            }
            frame #2 {
              n430 = while {
                stop <- w621 stop-if-true
                n431 = local read "Index ที่มากที่สุด"() -> (w624:i32)
                n432 = local read "commu"() -> (w619:T5)
                n433 = local read "Clear1"() -> (w620:bool)
                n434 = Equal?(x=w624, y=1) -> (x = y?=→"call":bool)
                n435 = Or(x=w619, y=w620) -> (x .or. y?=w621:T5)
              }
            }
            frame #3 {
              n436 = while {
                stop <- w625 stop-if-true
                n437 = local read "Index ที่มากที่สุด"() -> (w630:i32)
                n438 = local read "Clear1"() -> (w626:bool)
                n439 = local read "Emer"() -> (w627:bool)
                n440 = Equal?(x=w630, y=2) -> (x = y?=→"com":bool)
                n441 = Or(x=w627, y=w626) -> (x .or. y?=w625:bool)
              }
            }
          }
          n442 = local read "Clear1"() -> (w609:bool)
        }
        n443 = while {
          stop <- w590 stop-if-true
          n444 = local read "Tab Control"() -> (w600:T2)
          n445 = Equal?(x=w600, y=T2."TAB 2" ("Tab Control")) -> (x = y?=w608:bool)
          n446 = Equal?(x=w600, y=T2."TAB 3" ("Tab Control")) -> (x = y?=w607:bool)
          n447 = Equal?(x=w600, y=T2."TAB 4" ("Tab Control")) -> (x = y?=w606:bool)
          n448 = Equal?(x=w600, y=T2."TAB 5" ("Tab Control")) -> (x = y?=w596:bool)
          n449 = Equal?(x=w600, y=T2."TAB 6" ("Tab Control")) -> (x = y?=w595:bool)
          n450 = Equal?(x=w600, y=T2."TAB 7" ("Tab Control")) -> (x = y?=w592:bool)
          n451 = Or(x=w608, y=w607) -> (x .or. y?=w605:bool)
          n452 = Or(x=w607, y=w606) -> (x .or. y?=w604:bool)
          n453 = Or(x=w596, y=w595) -> (x .or. y?=w593:bool)
          n454 = Or(x=w605, y=w604) -> (x .or. y?=w594:bool)
          n455 = Or(x=w593, y=w592) -> (x .or. y?=w591:bool)
          n456 = Or(x=w594, y=w591) -> (x .or. y?=w590:bool)
          "Clear1" <- w590
        }
      }
    }
  }
  n457 = while {
    tunnel: w1 -> [w685]
    tunnel: [w684] -> w5
    tunnel: w4 -> [w683]
    tunnel: [w682] -> w3
    stop <- FALSE stop-if-true
    n458 = case shown="\"TAB 1\", Default" "Tab Control" {
      selector: "Tab Control" -> [w689 w713 w722 w731 w743 w753 w763]
      tunnel: [w688 w710 w719 w729 w739 w749 w759] -> w681
      frame "TAB 1", Default {
        n459 = local read "Index ที่มากที่สุด"() -> (w690:i32)
        n460 = local read "commu"() -> (w691:T5)
        n461 = Add(x=w689, y=3) -> (x+y=w708:u32)
        n462 = local read "Index ที่มากที่สุด"() -> (w696:i32)
        n463 = local read "ele"() -> (w695:T3)
        n464 = local read "Index ที่มากที่สุด"() -> (w694:i32)
        n465 = Equal?(x=w690, y=2) -> (x = y?=w706:bool)
        n466 = Increment(x=w689) -> (x+1=w700:T2)
        n467 = local read "call"() -> (w693:T4)
        n468 = And(x=w691, y=w706) -> (x .and. y?=w707:T5)
        n469 = Equal?(x=w696, y=0) -> (x = y?=w704:bool)
        n470 = Equal?(x=w694, y=1) -> (x = y?=w705:bool)
        n471 = And(x=w693, y=w705) -> (x .and. y?=w701:T4)
        n472 = And(x=w695, y=w704) -> (x .and. y?=w702:T3)
        n473 = Select(t=w708, s=w707, f=w689) -> (s? t:f=w709:u32)
        n474 = Select(t=w708, s=w701, f=w709) -> (s? t:f=w703:u32)
        n475 = Select(t=w700, s=w702, f=w703) -> (s? t:f=w688:u32)
      }
      frame "TAB 2" {
        n476 = local read "Index ที่มากที่สุด"() -> (w716:i32)
        n477 = local read "back_page2"() -> (w717:T7)
        n478 = Decrement(x=w713) -> (x-1=w715:T2)
        n479 = Equal?(x=w716, y=3) -> (x = y?=w712:bool)
        n480 = Not(x=w712) -> (.not. x?=w711:bool)
        n481 = And(x=w717, y=w712) -> (x .and. y?=w714:T7)
        n482 = local write "commu"(w711) -> ()
        n483 = Select(t=w715, s=w714, f=w713) -> (s? t:f=w710:T2)
      }
      frame "TAB 3" {
        n484 = local read "Index ที่มากที่สุด"() -> (w727:i32)
        n485 = local read "BACK_Page3"() -> (w724:bool)
        n486 = Subtract(x=w722, y=2) -> (x-y=w720:u32)
        n487 = Equal?(x=w727, y=3) -> (x = y?=w725:bool)
        n488 = And(x=w724, y=w725) -> (x .and. y?=w726:bool)
        n489 = Not(x=w725) -> (.not. x?=w723:bool)
        n490 = local write "call"(w723) -> ()
        n491 = Select(t=w720, s=w726, f=w722) -> (s? t:f=w719:u32)
      }
      frame "TAB 4" {
        n492 = local read "Index ที่มากที่สุด"() -> (w737:i32)
        n493 = local read "BACK_Page4"() -> (w734:bool)
        n494 = Subtract(x=w731, y=3) -> (x-y=w730:u32)
        n495 = Equal?(x=w737, y=3) -> (x = y?=w735:bool)
        n496 = And(x=w734, y=w735) -> (x .and. y?=w736:bool)
        n497 = Not(x=w735) -> (.not. x?=w733:bool)
        n498 = local write "ele"(w733) -> ()
        n499 = Select(t=w730, s=w736, f=w731) -> (s? t:f=w729:u32)
      }
      frame "TAB 5" {
        n500 = local read "BACK_Page5"() -> (w741:bool)
        n501 = local read "Index ที่มากที่สุด"() -> (w747:i32)
        n502 = Subtract(x=w743, y=3) -> (x-y=w742:u32)
        n503 = Equal?(x=w747, y=3) -> (x = y?=w745:bool)
        n504 = And(x=w741, y=w745) -> (x .and. y?=w746:bool)
        n505 = Not(x=w745) -> (.not. x?=w740:bool)
        n506 = local write "Emotion"(w740) -> ()
        n507 = Select(t=w742, s=w746, f=w743) -> (s? t:f=w739:u32)
      }
      frame "TAB 6" {
        n508 = local read "BACK_Page6"() -> (w751:T9)
        n509 = local read "Index ที่มากที่สุด"() -> (w757:i32)
        n510 = Subtract(x=w753, y=4) -> (x-y=w752:u32)
        n511 = Equal?(x=w757, y=3) -> (x = y?=w755:bool)
        n512 = And(x=w751, y=w755) -> (x .and. y?=w756:T9)
        n513 = Not(x=w755) -> (.not. x?=w750:bool)
        n514 = local write "Activity"(w750) -> ()
        n515 = Select(t=w752, s=w756, f=w753) -> (s? t:f=w749:u32)
      }
      frame "TAB 7" {
        n516 = local read "BACK_Page7"() -> (w761:bool)
        n517 = local read "Index ที่มากที่สุด"() -> (w767:i32)
        n518 = Subtract(x=w763, y=4) -> (x-y=w762:u32)
        n519 = Equal?(x=w767, y=3) -> (x = y?=w765:bool)
        n520 = And(x=w761, y=w765) -> (x .and. y?=w766:bool)
        n521 = Not(x=w765) -> (.not. x?=w760:bool)
        n522 = local write "ACC"(w760) -> ()
        n523 = Select(t=w762, s=w766, f=w763) -> (s? t:f=w759:u32)
      }
    }
    n524 = local write "Tab Control"(w681) -> ()
    n525 = Send Notification(notification=w681, notifier=w685, error in (no error)=w683) -> (notifier out=w684:refnum<notifier>, error out=w682:errorcluster)
  }
  n526 = while {
    shift-right: [w769] -> _
    shift-left: "" -> [w771]
    stop <- FALSE stop-if-true
    n527 = event shown="[2] \"Text3\": Value Change" {
      selector: _ -> [_ _ _ _]
      dyn-events: _ -> [_ _ _ _]
      timeout: _ -> [_ _ _ _]
      tunnel: w771 -> [_ _ _ w776]
      tunnel: ["Massage Send 2" "Massage Send 2" "Massage Send 3" w775] -> w769
      event "Text1": Value Change {
        n528 = event-data() -> ()  [unwired: 1 in, 6 out]
      }
      event Value Change {
        n529 = event-data() -> ()  [unwired: 1 in, 6 out]
      }
      event Value Change {
        n530 = event-data() -> ()  [unwired: 1 in, 6 out]
      }
      event "Clearpage 2": Value Change {
        n531 = event-data() -> ("CtlRef"=w778:refnum<vi>)  [unwired: 1 in, 3 out]
        n532 = property class="Bool (strict)"(reference=w778) -> ("Label.Text"=w777:string)  [unwired: 1 in, 2 out]
        n533 = case shown="\"Backspacepage 2\", Default" w777 {
          tunnel: w776 -> [w780 _]
          tunnel: [w779 ""] -> w775
          frame "Backspacepage 2", Default {
            n534 = String Length(string=w780) -> (length=w781:i32)
            n535 = Decrement(x=w781) -> (x-1=w782:i32)
            n536 = String Subset(string=w780, length (rest)=w782) -> (substring=w779:string)  [unwired: 1 in]
          }
          frame "Clearpage 2" {
          }
        }
      }
    }
    "Message Display" <- w769
  }
  n537 = Release Notifier(notifier=w5, error in (no error)=w3) -> ()  [unwired: 1 in, 3 out]
  n538 = call <vilib>:"Draw Flattened Pixmap.vi"() -> ()  [unwired: 9 in, 1 out]
  n539 = call <vilib>:"Draw Flattened Pixmap.vi"() -> ()  [unwired: 9 in, 1 out]
  n540 = call <vilib>:"Draw Flattened Pixmap.vi"() -> ()  [unwired: 9 in, 1 out]
